vi "ComplexCalculator.vi"() -> ()   [LabVIEW 2013]
panel:
  in  "InputData":T1(tab) caption="Dados de entrada"
  in  "jd":dbl[](array[numeric])
  in  "jb":dbl[](array[numeric])
  in  "c":dbl[](array[numeric])
  in  "a":dbl[](array[numeric])
  in  "Index":i32
  in  "InputFunction":T2(tab) caption="Operações matemáticas com complexos"
  in  "Simplificate":bool
  out "x":dbl
  out "jy":dbl
  out "z":dbl
  out "x 2":dbl caption="x"
  out "jy 2":dbl caption="jy"
  out "z 2":dbl caption="z"
  in  "CalculateModule":bool
  out "Módulo decimal":dbl
  out "Módulo fracionário":string
  in  "Representation":bool
  out "Exponential":string caption="Exponencial"
  out "Polar":string
  out "Trigonometric":string caption="Trigonométrica"
  # "Caso não haja alguma variável,\nbastapreencher com 0.\nCaso não haja denominador,\nmanter o numero real = 1"
  # "Formato do complexo:\n\n(a + jb)/(c + jd)"
  # "A"
  # "B"
  # "Seleciona o valor complexo referente ao\nrespectivo indice do vetor de entrada, e \nefetua os calculos desejados."
  # "Conjugado"
  # "Simplificação"
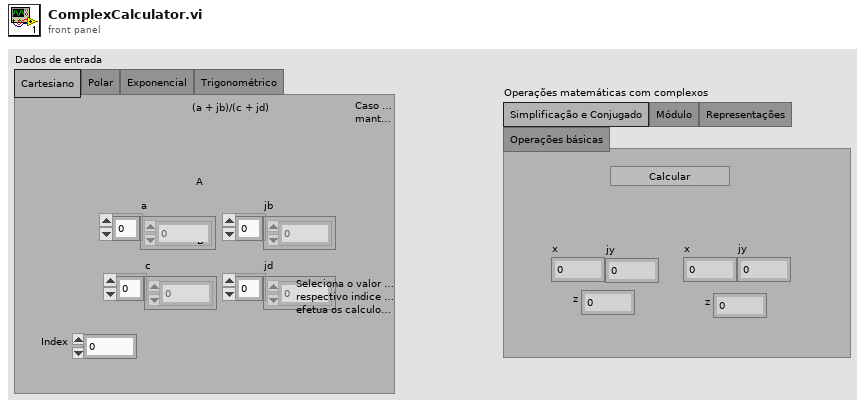
[diagram p1: front panel]
types:
  T1 = enum32{"Cartesiano", "Polar", "Exponencial", "Trigonométrico"}
  T2 = enum32{"Simplificação e Conjugado", "Módulo", "Representações", "Operações básicas"}
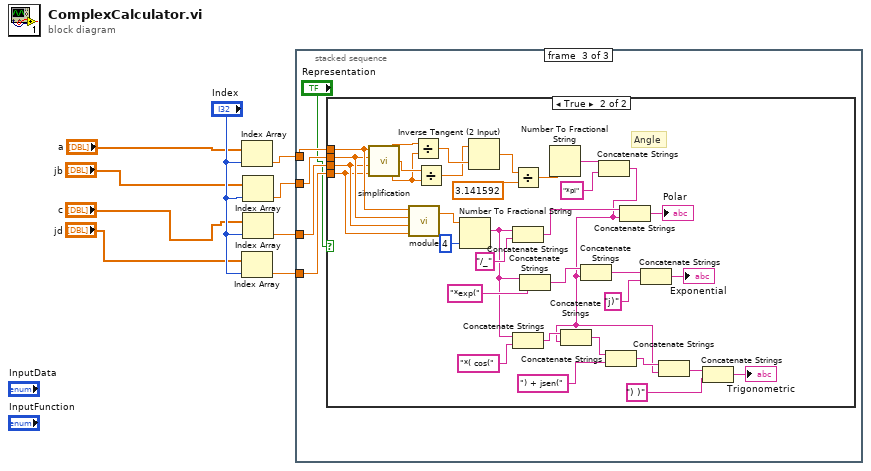
[diagram p0: block diagram]
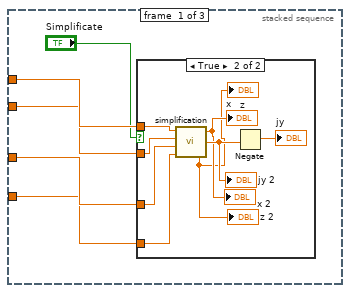
[diagram p2: hidden frame]
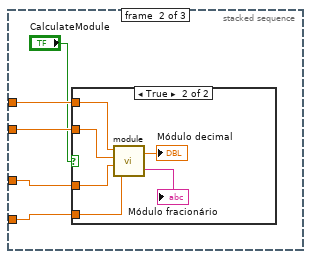
[diagram p4: hidden frame]
diagram:
  n1 = Index Array(array="a", index="Index") -> (element=w4:dbl)
  n2 = Index Array(array="jd", index="Index") -> (element=w1:dbl)
  n3 = Index Array(array="jb", index="Index") -> (element=w3:dbl)
  n4 = Index Array(array="c", index="Index") -> (element=w2:dbl)
  n5 = stacked-sequence {
    tunnel: w4 -> [w14 w27 w38]
    tunnel: w3 -> [w13 w26 w37]
    tunnel: w2 -> [w12 w25 w36]
    tunnel: w1 -> [w11 w24 w35]
    frame #0 {
      n6 = case shown="True" "Simplificate" {
        tunnel: w14 -> [_ w16]
        tunnel: w13 -> [_ w15]
        tunnel: w12 -> [_ w18]
        tunnel: w11 -> [_ w17]
        frame False {
        }
        frame True {
          n7 = call "simplification.vi"("jd"=w17, "c"=w18, "jb"=w15, "a"=w16) -> ("z"=→"z 2" →"z":dbl, "jy"=w22:dbl, "x"=→"x 2" →"x":dbl)
          "jy 2" <- w22
          n8 = Negate(x=w22) -> (-x=→"jy":dbl)
        }
      }
    }
    frame #1 {
      n9 = case shown="True" "CalculateModule" {
        tunnel: w27 -> [_ w33]
        tunnel: w26 -> [_ w32]
        tunnel: w25 -> [_ w31]
        tunnel: w24 -> [_ w30]
        frame False {
        }
        frame True {
          n10 = call "module.vi"("jd"=w30, "c"=w31, "jb"=w32, "a"=w33) -> ("Módulo fracionário"=→"Módulo fracionário":string, "Módulo decimal"=→"Módulo decimal":dbl)
        }
      }
    }
    frame #2 {
      n11 = case shown="True" "Representation" {
        tunnel: w38 -> [_ w62]
        tunnel: w37 -> [_ w61]
        tunnel: w36 -> [_ w60]
        tunnel: w35 -> [_ w59]
        frame False {
        }
        frame True {
          # "Angle"
          n12 = call "simplification.vi"("jd"=w59, "c"=w60, "jb"=w61, "a"=w62) -> ("z"=w70:dbl, "jy"=w71:dbl, "x"=w72:dbl)
          n13 = call "module.vi"("jd"=w59, "c"=w60, "jb"=w61, "a"=w62) -> ("Módulo decimal"=w58:dbl)  [unwired: 1 out]
          n14 = Divide(x=w72, y=w70) -> (x/y=w69:dbl)
          n15 = Divide(x=w71, y=w70) -> (x/y=w68:dbl)
          n16 = Number To Fractional String(number=w58, precision (6)=i16 4) -> (F-format string=w47:string)  [unwired: 2 in]
          n17 = Inverse Tangent (2 Input)(1:w69, 2:w68) -> (0:w67:dbl)
          n18 = Divide(x=w67, y=3.141592) -> (x/y=w65:dbl)
          n19 = Concatenate Strings(w47, "/_") -> (w55:string)
          n20 = Concatenate Strings(w47, "*( cos(") -> (w46:string)
          n21 = Concatenate Strings(w47, "*exp(") -> (w52:string)
          n22 = Number To Fractional String(number=w65) -> (F-format string=w64:string)  [unwired: 3 in]
          n23 = Concatenate Strings(w64, "*pi") -> (w42:string)
          n24 = Concatenate Strings(w46, w42) -> (w45:string)
          n25 = Concatenate Strings(w52, w42) -> (w51:string)
          n26 = Concatenate Strings(w45, ") + jsen(") -> (w43:string)
          n27 = Concatenate Strings(w55, w42) -> (→"Polar":string)
          n28 = Concatenate Strings(w51, "j)") -> (→"Exponential":string)
          n29 = Concatenate Strings(w43, w42) -> (w41:string)
          n30 = Concatenate Strings(w41, ") )") -> (→"Trigonometric":string)
        }
      }
    }
  }
